vi "make_waveform.vi"(8 "error in":errorcluster, 11 "Resonance Curve Data in":refnum<class "Resonance Curve Data.lvclass">) -> (0 "error out":errorcluster, 2 "2D waveform out":T1(array[cluster]), 3 "Resonance Curve Data out":refnum<class "Resonance Curve Data.lvclass">)   [LabVIEW 2020, in "Resonance Curve Data.lvclass"]
uses:
  Resonance Curve Data.lvclass
  Resonance Curve Data.lvclass/Resonance Curve Data.ctl
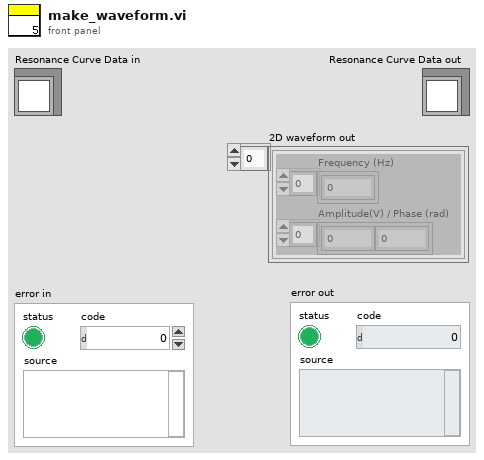
[diagram p1: front panel]
types:
  T1 = cluster{"Frequency (Hz)":dbl[], "Amplitude(V) / Phase (rad)":dbl[]}[]
  T2 = cluster{"Frequency (Hz)":dbl[], "Amplitude(V) / Phase (rad)":dbl[]}
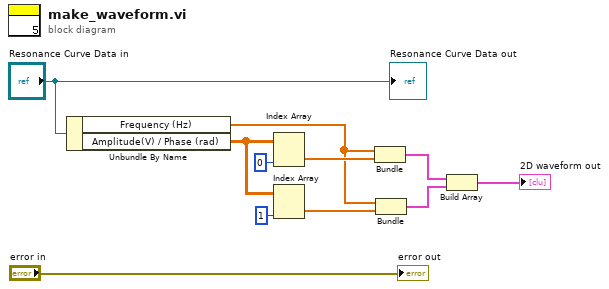
[diagram p0: block diagram]
diagram:
  n1 = Unbundle By Name("Resonance Curve Data in") -> ("Frequency (Hz)"=w5:dbl[], "Amplitude(V) / Phase (rad)"=w10:dbl[][])
  n2 = Index Array(array=w10, index (col)=0) -> (element=w7:dbl[])  [unwired: 1 in]
  n3 = Index Array(array=w10, index (col)=1) -> (element=w6:dbl[])  [unwired: 1 in]
  n4 = Bundle("Frequency (Hz)"=w5, "Amplitude(V) / Phase (rad)"=w7) -> (w4:T2)  [unwired: 1 in]
  n5 = Bundle("Frequency (Hz)"=w5, "Amplitude(V) / Phase (rad)"=w6) -> (w3:T2)  [unwired: 1 in]
  n6 = Build Array(w4, w3) -> (→"2D waveform out":T1)
  "Resonance Curve Data out" <- "Resonance Curve Data in"
  "error out" <- "error in"
